vi "Acquire Image.vi"(8 "Error In":errorcluster, 10 "File Path":path, 11 "Acquisition Memory":T1[](array[typedef])) -> (0 "Error Out":errorcluster, 2 "Source Image":T1, 3 "Pre-processed Image":T1, 5 "histogram":u32[](array[numeric]))   [LabVIEW 2018]
uses:
  <vilib>/vision/Image Controls.llb/IMAQ Image.ctl
  <vilib>/vision/NI_Vision_Development_Module.lvlib
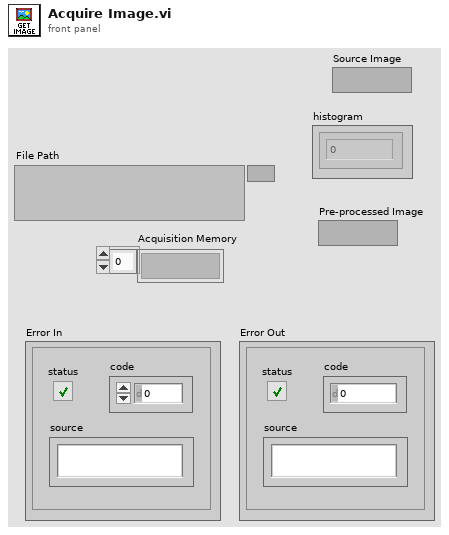
[diagram p1: front panel]
types:
  T1 = typedef "IMAQ Image.ctl" = refnum<image>
  T2 = typedef "Image Type" = u32
  T3 = cluster{"histogram":u32[], "Minimal Value":sgl, "Maximal Value":sgl, "Starting Value":sgl, "Interval Width":sgl, "Mean Value":sgl, "Standard  Variation":sgl, "Area (pixels)":i32}
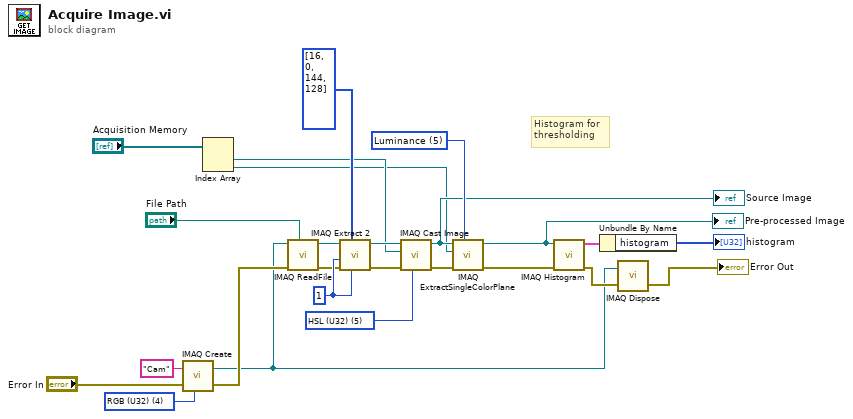
[diagram p0: block diagram]
diagram:
  w8 = 5 items=["Red", "Green", "Blue", "Hue", "Saturation", "Luminance", "Value", "Intensity"] ("Color Plane")
  w13 = T2 5 items=["Grayscale (U8)", "Grayscale (I16)", "Grayscale (SGL)", "Complex (CSG)", "RGB (U32)", "HSL (U32)", "RGB (U64)", "Grayscale (U16)"] ("Image Type")
  w16 = T2 4 items=["Grayscale (U8)", "Grayscale (I16)", "Grayscale (SGL)", "Complex (CSG)", "RGB (U32)", "HSL (U32)", "RGB (U64)", "Grayscale (U16)"] ("Image Type")
  w24 = 1 ("Y Step Size")
  # "Histogram for\nthresholding"
  n1 = call "IMAQ Create"("Image Name"="Cam", "Image Type"=w16, "error in (no error)"="Error In") -> ("New Image"=w6:T1, "error out"=w18:errorcluster)  [unwired: 2 in]
  n2 = Index Array(array="Acquisition Memory") -> (element #1=w5:T1, element #2=w3:T1)  [unwired: 2 in]
  n3 = call "IMAQ ReadFile"("File Path"="File Path", "error in (no error)"=w18, "Image"=w6) -> ("error out"=w12:errorcluster, "Image Out"=w11:T1)  [unwired: 4 in, 3 out]
  n4 = call "IMAQ Extract 2"("Y Step Size"=w24, "Optional Rectangle"=i32[] [16, 0, 144, 128], "error in (no error)"=w12, "X Step Size"=w24, "Image Src"=w11) -> ("error out"=w7:errorcluster, "Image Dst Out"=w10:T1)  [unwired: 5 in]
  n5 = call "IMAQ Cast Image"("Image Type"=w13, "error in (no error)"=w7, "Image Dst"=w5, "Image Src"=w10) -> ("error out"=w9:errorcluster, "Image Dst Out"=w4:T1)  [unwired: 6 in]
  "Source Image" <- w4
  n6 = call "IMAQ ExtractSingleColorPlane"("Color Plane"=w8, "error in (no error)"=w9, "Image Dst"=w3, "Image Src"=w4) -> ("error out"=w1:errorcluster, "Image Dst Out"=w2:T1)  [unwired: 6 in]
  "Pre-processed Image" <- w2
  n7 = call "IMAQ Histogram"("error in (no error)"=w1, "Image"=w2) -> ("error out"=w17:errorcluster, "Histogram Report"=w22:T3)  [unwired: 8 in]
  n8 = Unbundle By Name(w22) -> ("histogram"=→"histogram":u32[])
  n9 = call "IMAQ Dispose"("Image"=w6, "error in (no error)"=w17) -> ("error out"=→"Error Out":errorcluster)  [unwired: 4 in]
